vi "Accelerometer Logger SPI.vi"() -> ()   [LabVIEW 2013]
uses:
  <vilib>/ni845x/ni845x.llb/ni845xControl.ctl
  I2C/Accelerometer Data.ctl
  <vilib>/Platform/TimedLoop/XDataNode/timing_clust.ctl
  <vilib>/Platform/TimedLoop/XDataNode/nitl_modes.ctl
  <vilib>/Platform/TimedLoop/XDataNode/wakeup.ctl
  <vilib>/Analysis/_algsub.llb/Real Vector Norm.vi
  <vilib>/platform/TimedLoop/XDataNode/XDataNode.xnode
  h5logger/h5logger.lvlib
  <vilib>/Platform/TimedLoop/XDataNode/XDNodeRunTimeDep.lvlib
  <vilib>/Analysis/NI_AALPro.lvlib
panel:
  out "Good":bool caption="Good connection"
  out "accel self test":dbl[](array[numeric])
  out "gyro self test":dbl[](array[numeric])
  out "whoami":u8 caption="Should be 0x71:" format="%.0x"
  in  "block size":i32=100
  out "actrate":dbl[unit] caption="Actual rate"
  out "Trigger":bool
  out "Gyro":waveform(dbl)[](graph)
  out "Accel":waveform(dbl)[](graph)
  out "# in queue":i32
  out "num tries":i32 caption="Number of retries"
  out "file":path caption="File name:"
  in  "Stop on trigger":bool=TRUE
  in  "zero":bool
  in  "Post trigger":dbl[unit]=0.5
  in  "Stop":bool
  in  "accel range (g)":u16(ring)=2 items=["2"=2, "4"=4, "8"=8, "16"=16]
  in  "gyro range (deg/sec)":u16(ring)=250 items=["250"=250, "500"=500, "1000"=1000, "2000"=2000]
  in  "Sampling rate":dbl[unit]=200.0
  # "Debug stuff:"
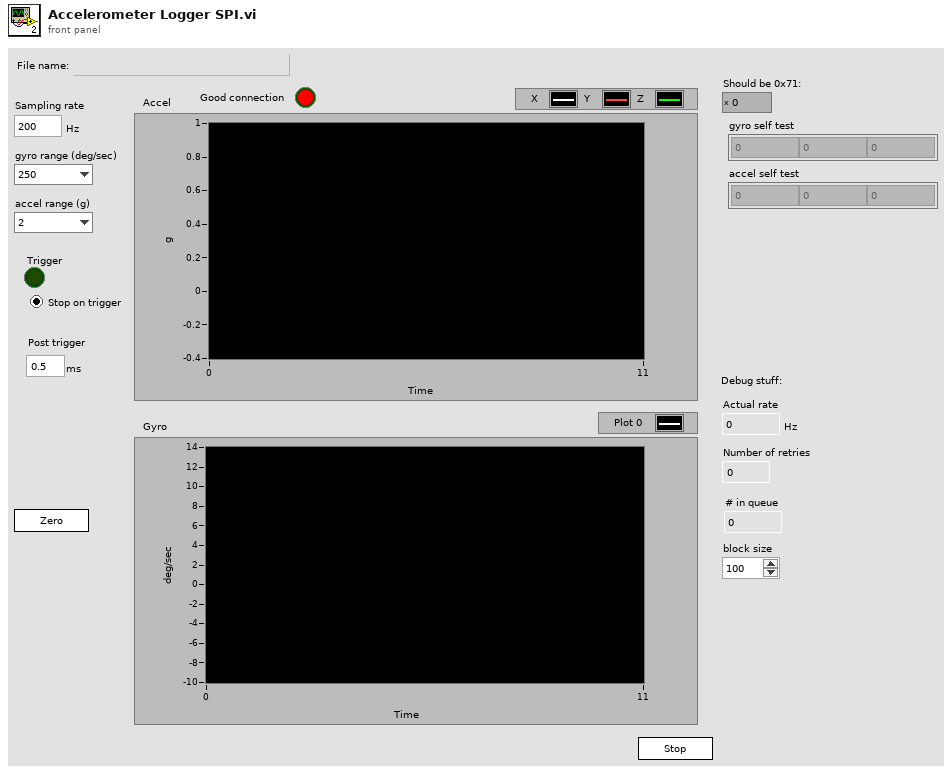
[diagram p1: front panel]
types:
  T1 = typedef "Accelerometer Data.ctl" = cluster{"Accel":dbl[], "Gyro":dbl[], "Time":u64, "Trigger":bool}
  T2 = typedef "ni845xControl.ctl" = refnum<k21>
  T3 = typedef "H5refs.ctl" = cluster{"File ref":T4, "t":i32, "accel":i32, "gyro":i32, "trigger":i32, "zero":i32}
  T4 = typedef "hid_t.ctl" = i32
  T5 = typedef "AccelerometerSPI.ctl" = cluster{"Device":T2, "spi configuration":T6}
  T6 = typedef "ni845xSpiConfiguration.ctl" = refnum<k20>
  T7 = typedef "XDNodeRunTimeDep.lvlib/timing_clust.ctl" = cluster{"Expected End [f-1]":u64, "Actual End [f-1]":u64, "Finished Late? [f-1]":bool, "Expected End [i-1]":u64, "Actual End [i-1]":u64, "Finished Late? [i-1]":bool, "Expected Start [i]":u64, "Actual Start [i]":u64, "Expected Start [f]":u64, "Actual Start [f]":u64, "Source Name":string, "Structure Name":string, "Period":i64, "Deadline":i64, "Offset":i64, "Start":i64, "Priority":i32, "Timeout":i32, "Mode":T8, "Wakeup Reason":T9, "Error":errorcluster, "Source Type":string, "Secondary Source Type":string, "Global End Time":u64, "Global Start Time":u64, "Frame Duration":u64, "Iteration Duration":u64, "Assigned CPU":i32, "I/O Scan Engine Mode":u32}
  T8 = typedef "XDNodeRunTimeDep.lvlib/nitl_modes.ctl" = enum32{"No Change", "Process missed periods, maintain original phase", "Discard missed periods, maintain original phase", "Process missed periods, ignore original phase", "Discard missed periods, ignore original phase"}
  T9 = typedef "XDNodeRunTimeDep.lvlib/wakeup.ctl" = enum32{"Normal", "Aborted", "Asynchronous wakeup", "Timing source error", "Timed loop error", "Timeout"}
  T10 = typedef "Accelerometer Data Block.ctl" = cluster{"Accel":dbl[][], "Gyro":dbl[][], "Time":u64[], "Trigger":bool[], "Zero":bool[]}
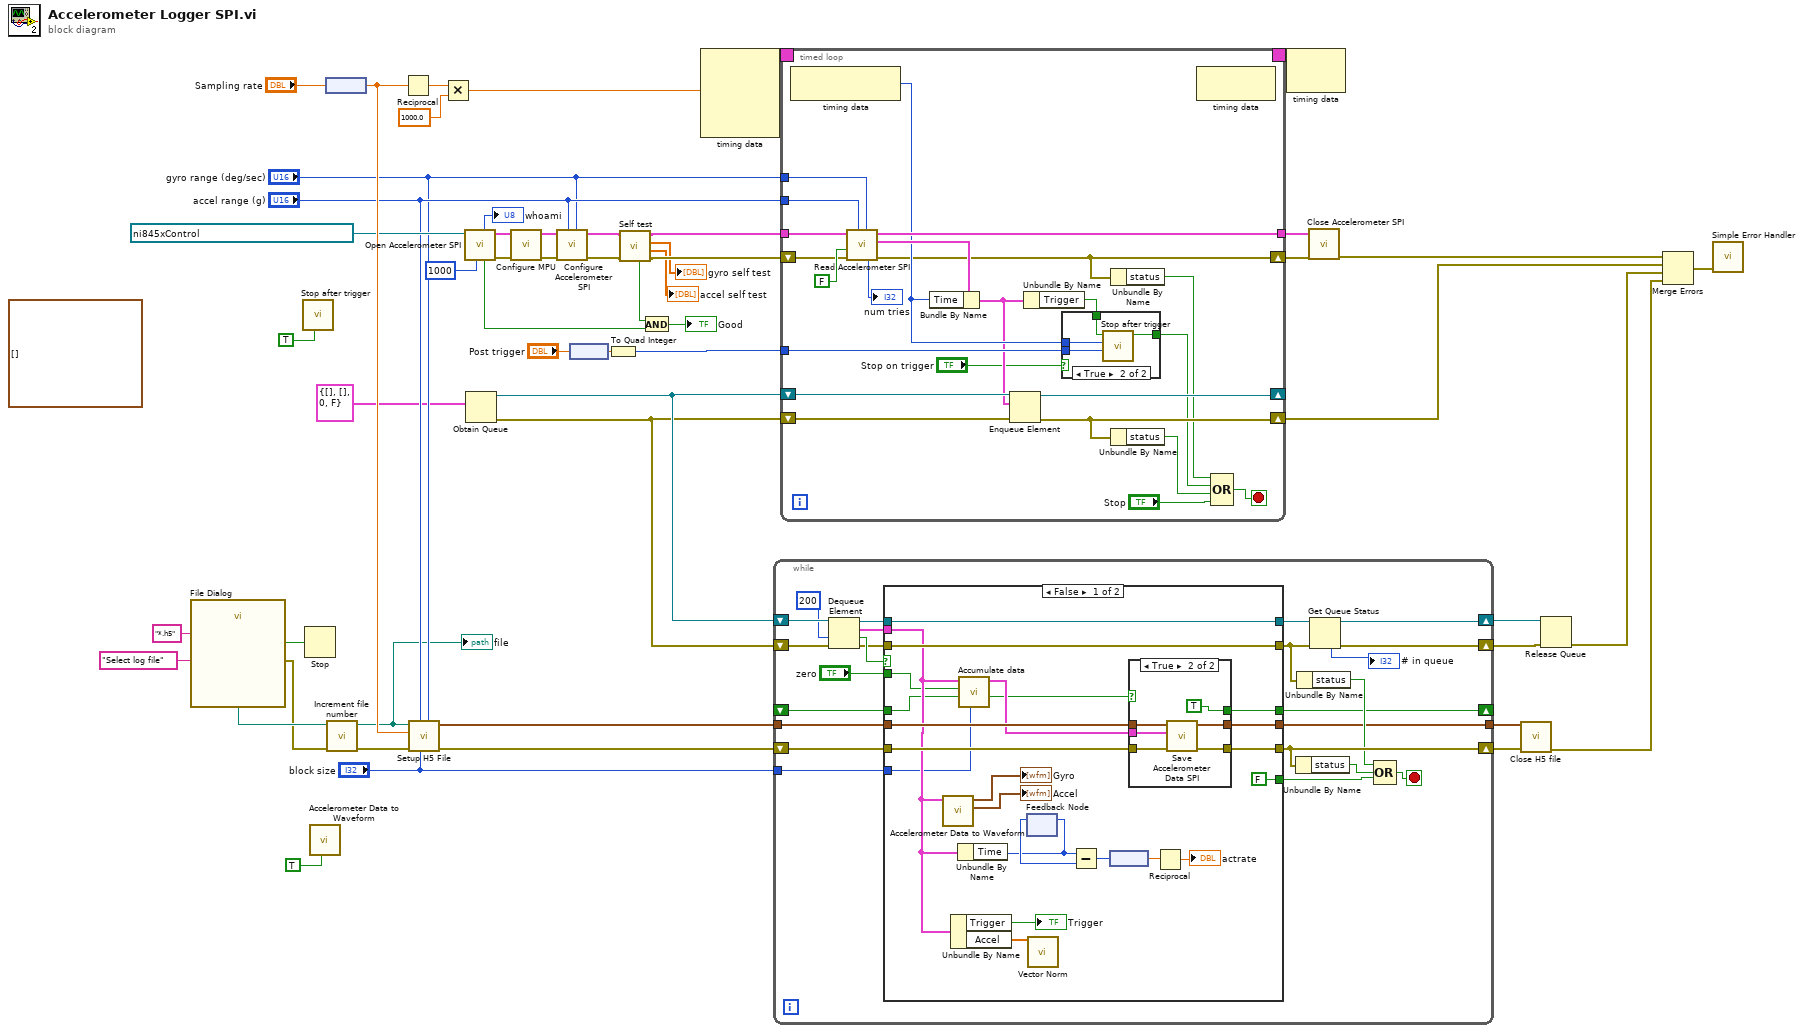
[diagram p0: block diagram]
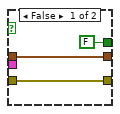
[diagram p2: hidden frame]
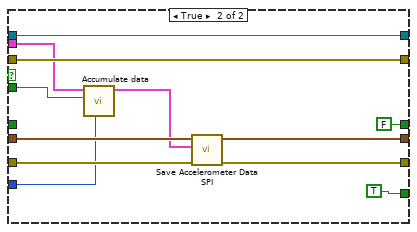
[diagram p3: hidden frame]
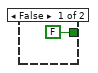
[diagram p4: hidden frame]
diagram:
  (unwired) waveform(dbl)[][] [] ("History Data")
  n1 = call "File Dialog"("prompt"="Select log file", "pattern (all files)"="*.h5") -> ("selected path"=w51:path, "cancelled"=w52:bool, "error out"=w50:errorcluster)  [unwired: 10 in, 1 out]
  n2 = call "Stop after trigger.vi"("reset"=TRUE) -> ()  [unwired: 10 in, 1 out]
  n3 = Stop(stop? (T)=w52) -> ()
  n4 = call "Accelerometer Data to Waveform.vi"("reset"=TRUE) -> ()  [unwired: 9 in, 2 out]
  n5 = node("Sampling rate") -> (w45:dbl)
  n6 = call "Increment file number.vi"("error in"=w50, "path"=w51) -> ("error out"=w49:errorcluster, "path out"=w19:path)  [unwired: 8 in]
  "file" <- w19
  n7 = Reciprocal(x=w45) -> (1/x=w44:dbl)
  n8 = call "Setup H5 File.vi"("Gyro range (deg/s)"="gyro range (deg/sec)", "block size"="block size", "Accel range (g)"="accel range (g)", "error in (no error)"=w49, "Sampling rate (Hz)"=w45, "path in"=w19) -> ("error out"=w22:errorcluster, "H5refs"=w33:T3)  [unwired: 4 in]
  n9 = Multiply(x=w44, y=1000.0) -> (x*y=w42:dbl)
  n10 = call "Open Accelerometer SPI.vi"("Clock Rate in kHz"=u16 1000, "Device"=T2 "USB0::0x3923::0x7166::01879089::RAW") -> ("error out"=w13:errorcluster, "Accelerometer"=w14:T5, "good"=w2:bool, "whoami"=→"whoami":u8)  [unwired: 6 in]
  n11 = Obtain Queue(element data type=T1 {"Accel"=[], "Gyro"=[], "Time"=0, "Trigger"=FALSE} ("Accelerometer Data")) -> (queue out=w18:refnum<queue>, error out=w17:errorcluster)  [unwired: 4 in, 1 out]
  n12 = call "Configure MPU.vi"("error in (no error)"=w13, "Accelerometer"=w14) -> ("error out"=w11:errorcluster, "Accelerometer out"=w12:T5)  [unwired: 8 in]
  n13 = call "Configure Accelerometer SPI.vi"("gyro range (deg/sec)"="gyro range (deg/sec)", "accel range (g)"="accel range (g)", "error in (no error)"=w11, "Accelerometer"=w12) -> ("error out"=w9:errorcluster, "Accelerometer out"=w10:T5)  [unwired: 6 in]
  n14 = node("Post trigger") -> (w35:dbl)
  n15 = To Quad Integer(1:w35) -> (0:w34:i64)
  n16 = call "Self test.vi"("error in (no error)"=w9, "Accelerometer"=w10) -> ("error out"=w7:errorcluster, "accel self test"=→"accel self test":dbl[], "gyro self test"=→"gyro self test":dbl[], "Accelerometer out"=w8:T5, "good"=w3:bool)  [unwired: 5 in]
  n17 = And(x=w3, y=w2) -> (x .and. y?=→"Good":bool)
  n18 = node-c288(w42) -> (w47:T7)  [unwired: 3 in]
  n19 = while {
    tunnel: w33 -> [w75]
    shift-right: [w71] -> w29
    shift-left: w22 -> [w74]
    shift-right: [w64] -> w31
    shift-left: w17 -> [w69]
    tunnel: [w67] -> w30
    shift-right: [w63] -> w32
    shift-left: w18 -> [w78]
    shift-right: [w56] -> _
    shift-left: _ -> [w57]
    tunnel: "block size" -> [w55]
    stop <- w72 stop-if-true
    n20 = Dequeue Element(queue=w78, timeout in ms (-1)=200, error in (no error)=w69) -> (queue out=w77:refnum<queue>, element=w76:T1, timed out?=w61:bool, error out=w59:errorcluster)
    n21 = case shown="False" w61 {
      tunnel: w77 -> [w98 w122]
      tunnel: w76 -> [w85 w119]
      tunnel: w75 -> [w101 w117]
      tunnel: w74 -> [w100 w115]
      tunnel: [w99 w113] -> w71
      tunnel: "zero" -> [w83 w118]
      tunnel: [w98 w122] -> w65
      tunnel: [w97 w114] -> w67
      tunnel: [w96 w121] -> w60
      tunnel: w59 -> [w96 w121]
      tunnel: [FALSE TRUE] -> w58
      tunnel: w57 -> [w80 _]
      tunnel: [w81 FALSE] -> w56
      tunnel: w55 -> [w79 w111]
      frame False {
        n22 = call "Accelerometer Data to Waveform.vi"("Accelerometer Data"=w85) -> ("accel plot"=→"Accel":waveform(dbl)[], "gyro plot"=→"Gyro":waveform(dbl)[])  [unwired: 9 in]
        n23 = Unbundle By Name(w85) -> ("Trigger"=→"Trigger":bool, "Accel"=w86:dbl[])
        n24 = Unbundle By Name(w85) -> ("Time"=w87:u64)
        n25 = call "Accumulate data.vi"("block size"=w79, "reset"=w80, "zero"=w83, "Accelerometer Data"=w85) -> ("done"=w82:bool, "Accelerometer Data Block"=w84:T10)  [unwired: 5 in, 1 out]
        n26 = feedback #1() -> (w88:u64)  [unwired: 1 in]
        n27 = feedback-in #1(w87) -> ()
        n28 = call-poly <vilib>:"Vector Norm.vi"("Input Vector"=w86) -> ()  [unwired: 9 in, 2 out]
        n29 = Subtract(x=w87, y=w88) -> (x-y=w89:u64)
        n30 = node(w89) -> (w90:dbl[unit])
        n31 = case shown="True" w82 {
          tunnel: w101 -> [w103 w110]
          tunnel: w100 -> [w102 w109]
          tunnel: [w102 w108] -> w99
          tunnel: [w103 w107] -> w97
          tunnel: w84 -> [_ w106]
          tunnel: [FALSE TRUE] -> w81
          frame False {
          }
          frame True {
            n32 = call "Save Accelerometer Data SPI.vi"("error in (no error)"=w109, "Accelerometer Data Block"=w106, "H5refs"=w110) -> ("error out"=w108:errorcluster, "H5refs out"=w107:T3)  [unwired: 7 in]
          }
        }
        n33 = Reciprocal(x=w90) -> (1/x=→"actrate":dbl[unit])
      }
      frame True {
        n34 = call "Accumulate data.vi"("block size"=w111, "zero"=w118, "Accelerometer Data"=w119) -> ("Accelerometer Data Block"=w116:T10)  [unwired: 6 in, 2 out]
        n35 = call "Save Accelerometer Data SPI.vi"("error in (no error)"=w115, "Accelerometer Data Block"=w116, "H5refs"=w117) -> ("error out"=w113:errorcluster, "H5refs out"=w114:T3)  [unwired: 7 in]
      }
    }
    n36 = Unbundle By Name(w71) -> ("status"=w70:bool)
    n37 = Unbundle By Name(w60) -> ("status"=w68:bool)
    n38 = Get Queue Status(queue=w65, error in (no error)=w60) -> (queue out=w63:refnum<queue>, error out=w64:errorcluster, # elements in queue=→"# in queue":i32)  [unwired: 1 in, 5 out]
    n39 = Compound Arithmetic op=OR(w68, w70, w58) -> (w72:bool)
  }
  n40 = timed-loop {
    timing: w47 -> [_]
    timing-out: [_] -> w46
    tunnel: w8 -> [w144]
    tunnel: "accel range (g)" -> [w142]
    tunnel: "gyro range (deg/sec)" -> [w141]
    tunnel: [w140] -> w27
    tunnel: w34 -> [w133]
    shift-right: [w136] -> _
    shift-left: w18 -> [w138]
    shift-right: [w130] -> w16
    shift-left: w17 -> [w137]
    shift-right: [w131] -> w28
    shift-left: w7 -> [w143]
    stop <- w129 stop-if-true
    n41 = node-c288() -> (w134:i64)  [unwired: 1 in]
    n42 = call "Read Accelerometer SPI.vi"("gyro range (deg/sec)"=w141, "accel range (g)"=w142, "error in (no error)"=w143, "check ready"=FALSE, "Accelerometer"=w144) -> ("error out"=w131:errorcluster, "Accelerometer Data"=w139:T1, "Accelerometer out"=w140:T5, "num tries"=→"num tries":i32)  [unwired: 3 in]
    n43 = Bundle By Name(cluster=w139, "Time"=w134) -> (w132:T1)
    n44 = Enqueue Element(queue=w138, element=w132, error in (no error)=w137) -> (queue out=w136:refnum<queue>, error out=w130:errorcluster)  [unwired: 1 in, 1 out]
    n45 = Unbundle By Name(w132) -> ("Trigger"=w135:bool)
    n46 = case shown="True" "Stop on trigger" {
      tunnel: w135 -> [_ w150]
      tunnel: w134 -> [_ w149]
      tunnel: w133 -> [_ w148]
      tunnel: [FALSE ("done") w147] -> w126
      frame False {
      }
      frame True {
        n47 = call "Stop after trigger.vi"("delay after trigger"=w148, "current time"=w149, "trigger"=w150) -> ("done"=w147:bool)  [unwired: 8 in]
      }
    }
    n48 = Unbundle By Name(w131) -> ("status"=w125:bool)
    n49 = Unbundle By Name(w130) -> ("status"=w127:bool)
    n50 = node-c288() -> ()  [unwired: 1 in, 1 out]
    n51 = Compound Arithmetic op=OR(w125, w126, w127, "Stop") -> (w129:bool)
  }
  n52 = node-c288(w46) -> ()  [unwired: 1 out]
  n53 = call "Close Accelerometer SPI.vi"("error in (no error)"=w28, "Accelerometer"=w27) -> ("error out"=w26:errorcluster)  [unwired: 9 in]
  n54 = call "Close H5 file.vi"("error in (no error)"=w29, "H5refs"=w30) -> ("error out"=w24:errorcluster)  [unwired: 9 in]
  n55 = Release Queue(queue=w32, error in (no error)=w31) -> (error out=w25:errorcluster)  [unwired: 1 in, 2 out]
  n56 = Merge Errors(w26, w16, w25, w24) -> (w23:errorcluster)
  n57 = call <vilib>:"Simple Error Handler.vi"("error in (no error)"=w23) -> ()  [unwired: 4 in, 5 out]
